vi "RSMA Receiver - 1 Channel Modulation Config.vi"() -> ()   [LabVIEW 2022 SP3]
panel:
  out "Constellation Map 2":cdb[](graph)
  out "BER vs. Time":T1(graph)
  in  "SIC Amp":dbl(slide)=4.610619469026549 scale=1.0..5.0
  out "Number of bits":dbl[](array[numeric])
  out "Accuracy error":dbl[](array[numeric])
  out "Accumulated error":dbl[](array[numeric])
  out "Iterations":dbl format="%#_4g"
  out "Decoded message":string
  out "Constellation Map":cdb[](graph)
  in  "Decode M2?":bool
  in  "Tab Control":enum32{"USRP Parameters", "Rx Info", "BER"}(tab)
  in  "USRP ControledParameters":T2={"Active Antenna"="RX2", "Gain (dB)"=0.0, "Carrier Frequency"=2400000000.0, "IQ Rate"=2000000.0, "Active channels"="0"} {"IQ Rate" format="%#_6p"; "Carrier Frequency" format="%#_6p"; "Gain (dB)" format="%#_6f"}
  in  "Device selection":refnum<k15>="RIO0"
  in  "Trigger level":dbl=0.01 format="%f"
  in  "Modulation 2":T3(ring)
  in  "Common Bits":i32=4
  in  "Total Bits":i32=6
  out "?":T4
  out "SIG valid?":bool
  out "Frequency offset":dbl
  out "Coerced Parameters":T5={"IQ Rate"=100000.0, "Carrier  Freq."=100000.0, "Gain"=0.0} {"Gain" format="%#_6f"; "Carrier  Freq." format="%#_6p"; "IQ Rate" format="%#_6p"}
  out "Error out":errorcluster
  in  "Expected message":string="Lorem ipsum dolor sit amet, consetetur sadipscing elitr, sed diam nonumy eirmod tempor invidunt ut labore et dolore magna aliquyam erat, sed diam volu"
  in  "Record BER":bool
  in  "Refresh Button":bool
  out "Inst. BER":dbl format="%#_4g"
  out "No. Bits":dbl format="%#_6f"
  out "Acum. Err":dbl
  out "Acc. BER":dbl format="%#_4g"
  in  "error in (no error)":errorcluster
  # "RSMA Reciever"
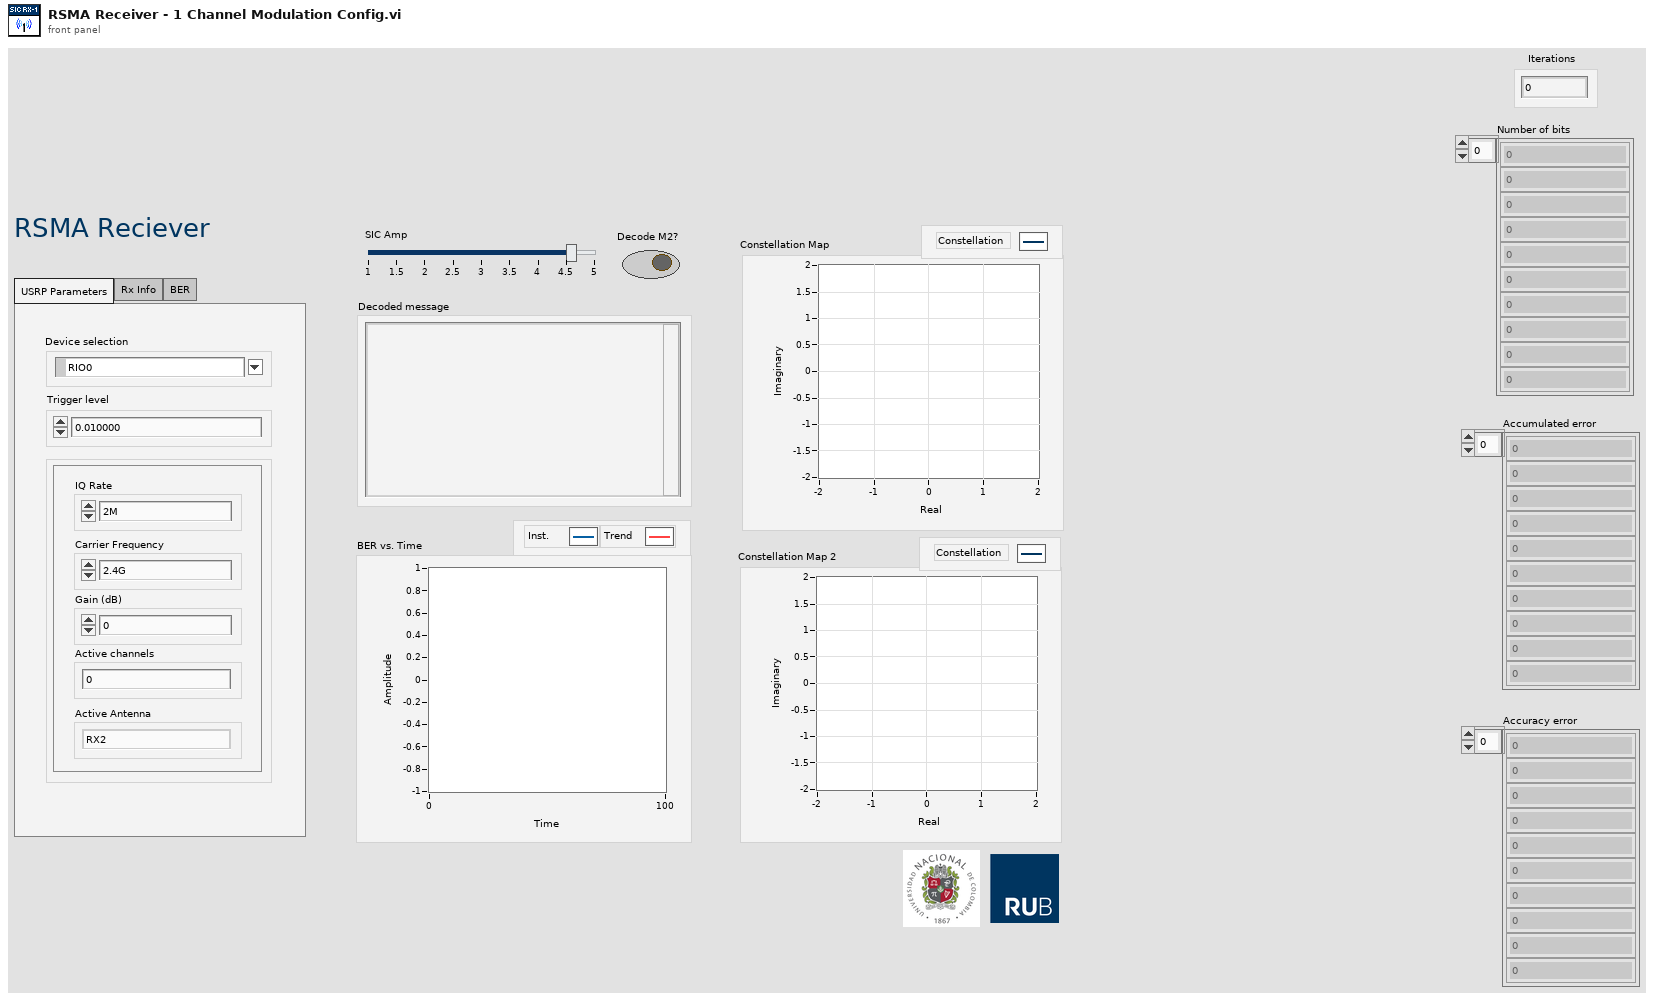
[diagram p1: front panel]
types:
  T1 = cluster{"Graph Instantaneous BER":dbl, "Graph Instantaneous BER":dbl}
  T2 = cluster{"Active Antenna":string, "Gain (dB)":dbl, "Carrier Frequency":dbl, "IQ Rate":dbl, "Active channels":string}
  T3 = enum16{"QPSK(4QAM)", "64QAM", "16QAM", "BPSK", "BPSK Vertical"}
  T4 = cluster{"Modulation type":enum16{"QPSK(4QAM)", "64QAM", "16QAM", "BPSK"}, "BCC rate (k/n)":enum16{"1/2", "2/3", "3/4"}}
  T5 = cluster{"IQ Rate":dbl, "Carrier  Freq.":dbl, "Gain":dbl}
  T6 = cluster{"coerced IQ rate":dbl, "coerced carrier frequency":dbl, "coerced gain":dbl}
  T7 = cluster{"Modulation type":enum16{"QPSK(4QAM)", "64QAM", "16QAM", "BPSK", "BPSK Vertical"}, "BCC rate (k/n)":enum16{"1/2", "2/3", "3/4"}}
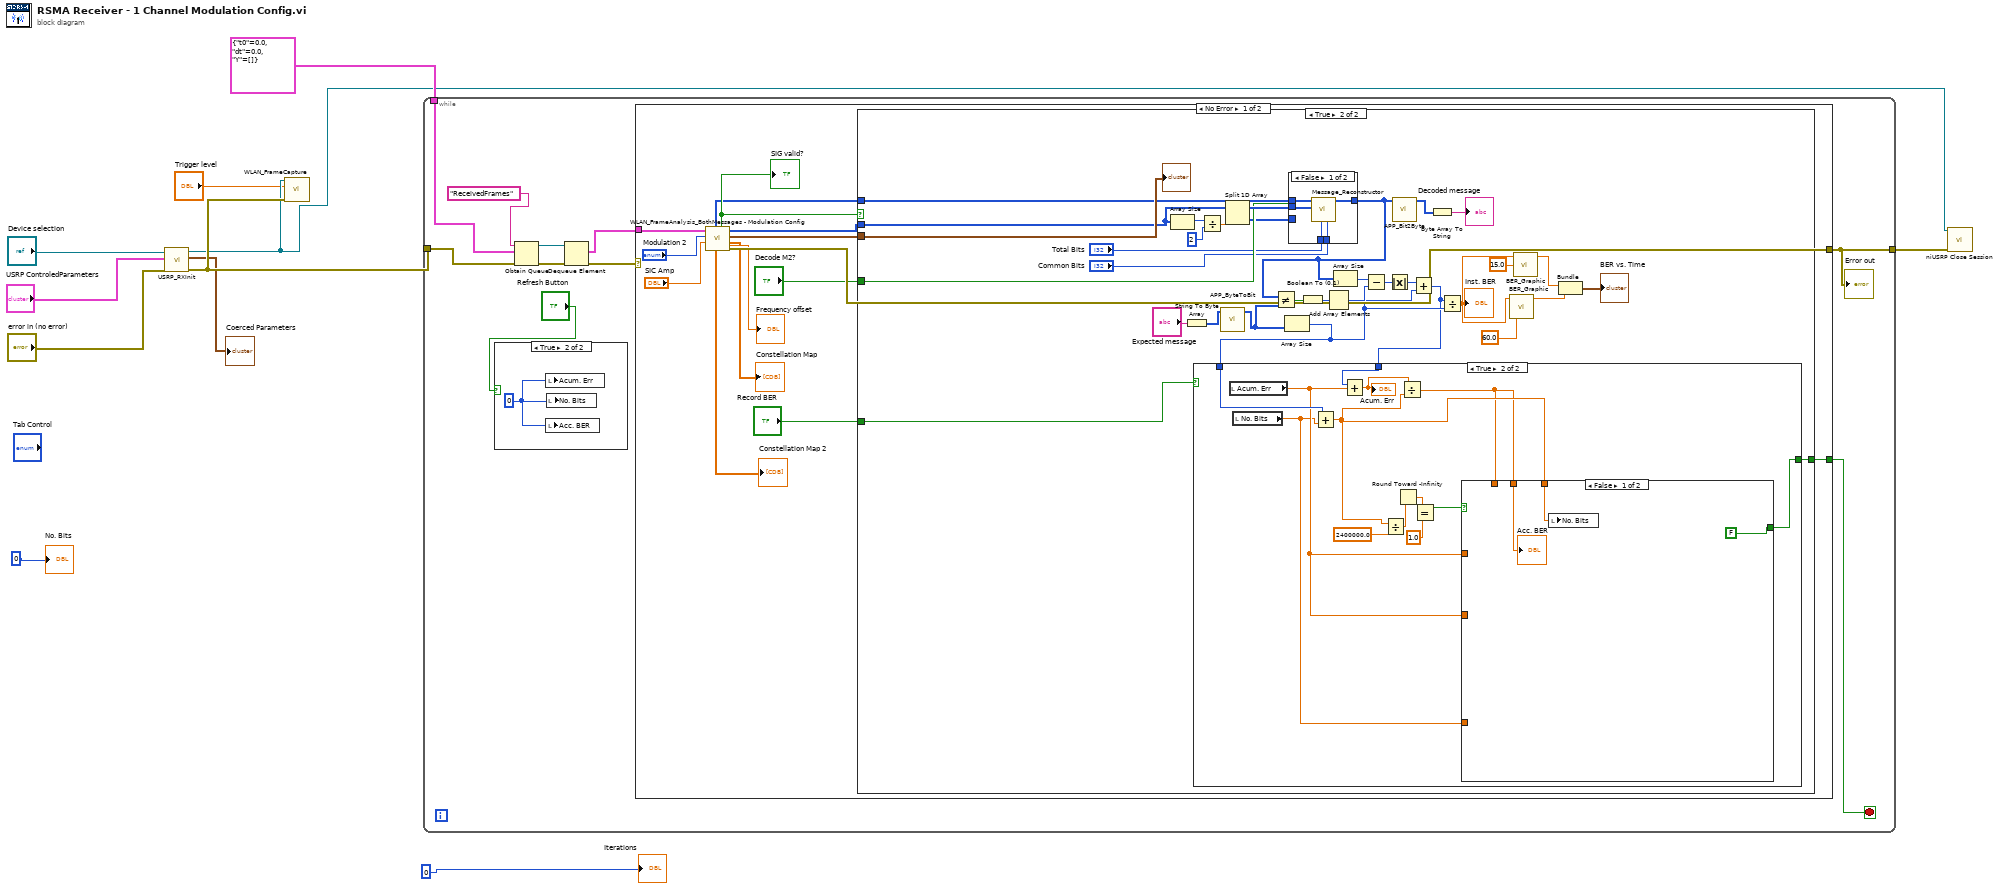
[diagram p0: block diagram]
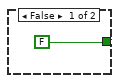
[diagram p3: hidden frame]
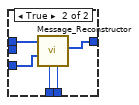
[diagram p4: hidden frame]
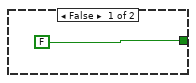
[diagram p5: hidden frame]
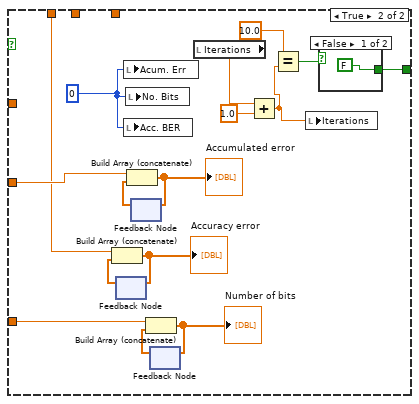
[diagram p6: hidden frame]
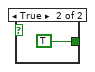
[diagram p7: hidden frame]
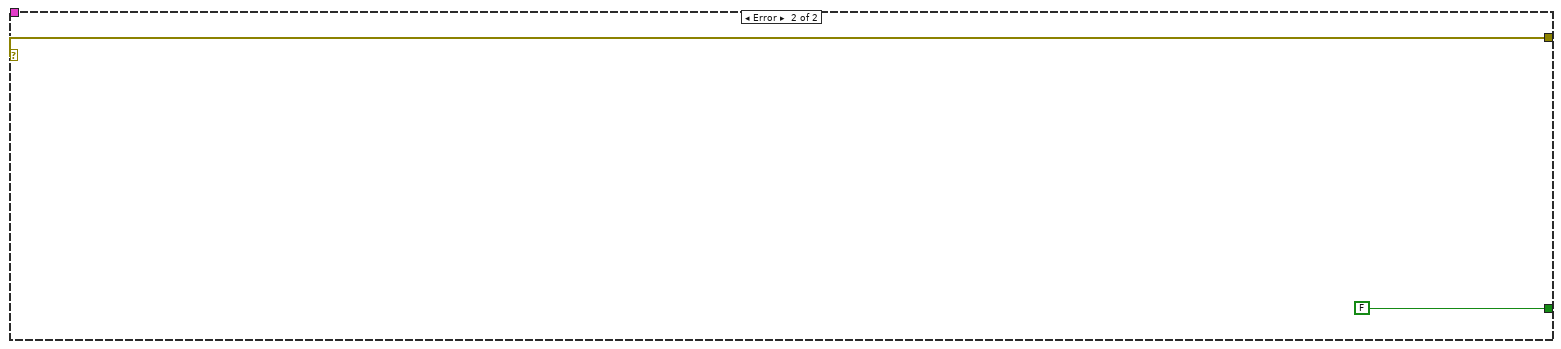
[diagram p8: hidden frame]
diagram:
  n1 = call "USRP_RXInit.vi"("device names"="Device selection", "USRP ControledParameters"="USRP ControledParameters", "error in (no error)"="error in (no error)") -> ("session handle out"=w7:refnum<k15>, "USRP CoercedParamters"=→"Coerced Parameters":T6, "error out"=w10:errorcluster)  [unwired: 5 in]
  n2 = call "WLAN_FrameCapture.vi"("error in (no error)"=w10, "Trigger level"="Trigger level", "session handle"=w7) -> ()  [unwired: 8 in]
  n3 = while {
    tunnel: w10 -> [w20]
    tunnel: cluster{"t0":dbl, "dt":dbl, "Y":cdb[]} {"t0"=0.0, "dt"=0.0, "Y"=[]} ("data") -> [w21]
    tunnel: [w14] -> w8
    stop <- w12 stop-if-true
    n4 = case shown="True" "Refresh Button" {
      frame False {
      }
      frame True {
        w22 = 0
        n5 = local write "Acum. Err"(w22) -> ()
        n6 = local write "Acc. BER"(w22) -> ()
        n7 = local write "No. Bits"(w22) -> ()
      }
    }
    n8 = Obtain Queue(name (unnamed)="ReceivedFrames", element data type=w21, error in (no error)=w20) -> (queue out=w19:refnum<queue>, error out=w16:errorcluster)  [unwired: 2 in, 1 out]
    n9 = Dequeue Element(queue=w19, error in (no error)=w16) -> (element=w17:cluster{"t0":dbl, "dt":dbl, "Y":cdb[]}, error out=w18:errorcluster)  [unwired: 1 in, 2 out]
    n10 = case shown="No Error" w18 {
      selector: w18 -> [_ w117]
      tunnel: w17 -> [w34 _]
      tunnel: [w35 w117] -> w14
      tunnel: [w26 FALSE] -> w12
      frame No Error {
        n11 = call "WLAN_FrameAnalysis_BothMessages - Modulation Config.vi"("SIC Amp"="SIC Amp", "Modulation 2"="Modulation 2", "input cluster"=w34) -> ("error out"=w35:errorcluster, "Constellation"=→"Constellation Map":cdb[], "Modulation parameter"=w36:T7, "SC Bits"=w28:i8[], "Frequency offset"=→"Frequency offset":dbl, "SIG valid?"=w33:bool, "Constellation 2"=→"Constellation Map 2":cdb[], "Base Bits"=w29:i8[])  [unwired: 1 in]
        "SIG valid?" <- w33
        n12 = case shown="True" w33 {
          tunnel: w36 -> [_ w70]
          tunnel: "Record BER" -> [_ w65]
          tunnel: w29 -> [_ w53]
          tunnel: w28 -> [_ w49]
          tunnel: "Decode M2?" -> [_ w52]
          tunnel: [FALSE w48] -> w26
          frame False {
          }
          frame True {
            n13 = Array Size(array=w49) -> (size(s)=w55:i32)
            n14 = String To Byte Array(string="Expected message") -> (unsigned byte array=w64:u8[])
            n15 = Divide(x=w55, y=2) -> (x/y=w56:dbl)
            n16 = call "APP_ByteToBit.vi"("byte array"=w64) -> ("bit array"=w63:i8[])  [unwired: 9 in]
            n17 = Split 1D Array(array=w49, index=w56) -> (first subarray=w54:i8[], second subarray=w51:i8[])
            n18 = Array Size(array=w63) -> (size(s)=w59:i32)
            n19 = case shown="False" w52 {
              tunnel: [w75 w78] -> w46
              tunnel: w54 -> [w74 _]
              tunnel: w53 -> [w73 w79]
              tunnel: w51 -> [_ w80]
              tunnel: "Total Bits" -> [w72 w77]
              tunnel: "Common Bits" -> [w71 w76]
              frame False {
                n20 = call "Message_Reconstructor.vi"("No. Common Bits"=w71, "No. Total Bits"=w72, "Wp1"=w74, "Wc"=w73) -> ("W1"=w75:u8[])  [unwired: 6 in, 1 out]
              }
              frame True {
                n21 = call "Message_Reconstructor.vi"("No. Common Bits"=w76, "No. Total Bits"=w77, "Wp2"=w80, "Wc"=w79) -> ("W2"=w78:u8[])  [unwired: 6 in, 1 out]
              }
            }
            n22 = Not Equal?(x=w46, y=w63) -> (x != y?=w67:bool[])
            n23 = Boolean To (0,1)(Boolean=w67) -> (0, 1=w66:i16[])
            n24 = Add Array Elements(numeric array=w66) -> (sum=w58:i16)
            n25 = Array Size(array=w46) -> (size(s)=w62:i32)
            n26 = Subtract(x=w62, y=w59) -> (x-y=w61:i32)
            n27 = Absolute Value(x=w61) -> (abs(x)=w60:i32)
            n28 = call "APP_Bit2Byte.vi"("input bit stream"=w46) -> ("output byte stream"=w47:u8[])  [unwired: 10 in]
            n29 = Add(x=w60, y=w58) -> (x+y=w57:i32)
            n30 = case shown="True" w65 {
              tunnel: w59 -> [_ w94]
              tunnel: w57 -> [_ w93]
              tunnel: [FALSE w85] -> w48
              frame False {
              }
              frame True {
                n31 = local read "Acum. Err"() -> (w84:dbl)
                n32 = local read "No. Bits"() -> (w82:dbl)
                n33 = Add(x=w94, y=w82) -> (x+y=w88:dbl)
                n34 = Add(x=w93, y=w84) -> (x+y=w92:dbl)
                "Acum. Err" <- w92
                n35 = Divide(x=w88, y=2400000.0) -> (x/y=w87:dbl)
                n36 = Round Toward -Infinity(1:w87) -> (0:w86:dbl)
                n37 = Divide(x=w92, y=w88) -> (x/y=w83:dbl)
                n38 = Equal?(x=w86, y=1.0) -> (x = y?=w89:bool)
                n39 = case shown="False" w89 {
                  tunnel: w84 -> [_ _]
                  tunnel: w88 -> [w97 _]
                  tunnel: w83 -> [w96 _]
                  tunnel: [FALSE w108] -> w85
                  tunnel: w84 -> [_ w106]
                  tunnel: w83 -> [_ w101]
                  tunnel: w82 -> [_ w98]
                  frame False {
                    n40 = local write "No. Bits"(w97) -> ()
                    "Acc. BER" <- w96
                  }
                  frame True {
                    w113 = 0
                    n41 = feedback #1() -> (w103:dbl[])  [unwired: 1 in]
                    n42 = Build Array (concatenate)(w101, w103) -> (w102:dbl[])
                    "Accuracy error" <- w102
                    n43 = feedback-in #1(w102) -> ()
                    n44 = local write "Acum. Err"(w113) -> ()
                    n45 = local write "Acc. BER"(w113) -> ()
                    n46 = local write "No. Bits"(w113) -> ()
                    n47 = feedback #2() -> (w105:dbl[])  [unwired: 1 in]
                    n48 = Build Array (concatenate)(w106, w105) -> (w104:dbl[])
                    "Accumulated error" <- w104
                    n49 = feedback-in #2(w104) -> ()
                    n50 = feedback #3() -> (w100:dbl[])  [unwired: 1 in]
                    n51 = Build Array (concatenate)(w98, w100) -> (w99:dbl[])
                    "Number of bits" <- w99
                    n52 = feedback-in #3(w99) -> ()
                    n53 = local read "Iterations"() -> (w112:dbl)
                    n54 = Add(x=w112, y=1.0) -> (x+y=w107:dbl)
                    n55 = Equal?(x=10.0, y=w107) -> (x = y?=w109:bool)
                    n56 = local write "Iterations"(w107) -> ()
                    n57 = case shown="False" w109 {
                      tunnel: [FALSE TRUE] -> w108
                      frame False {
                      }
                      frame True {
                      }
                    }
                  }
                }
              }
            }
            n58 = Byte Array To String(unsigned byte array=w47) -> (string=→"Decoded message":string)
            n59 = Divide(x=w57, y=w59) -> (x/y=w41:dbl)
            "Inst. BER" <- w41
            n60 = call "BER_Graphic.vi"("Window Size"=60.0, "Instantaneous BER"=w41) -> ("Graph Instantaneous BER"=w39:dbl)  [unwired: 3 in]
            n61 = call "BER_Graphic.vi"("Window Size"=15.0, "Instantaneous BER"=w41) -> ("Graph Instantaneous BER"=w40:dbl)  [unwired: 3 in]
            n62 = Bundle("Graph Instantaneous BER"=w40, "Graph Instantaneous BER"=w39) -> (→"BER vs. Time":T1)  [unwired: 1 in]
            "?" <- w70
          }
        }
      }
      frame Error {
      }
    }
    "Error out" <- w14
  }
  n63 = call <instrlib>:"niUSRP Close Session.vi"("session handle"=w7, "error in (no error)"=w8) -> ()  [unwired: 13 in, 1 out]
  "No. Bits" <- 0
  "Iterations" <- 0
